vi "Init Scene.vi"(8 "error in (no error)":errorcluster, 11 "SceneGraph Refnum":refnum<vi>) -> (0 "error out":errorcluster, 3 "Voronoi Grid Object":refnum<vi>)   [LabVIEW 2023]
doc: "Initialize the overall scene by setting camera parameters and creating the object for the Voronoi surface."
uses:
  <vilib>/Utility/miscctls.llb/LV3DPointTypeDef.ctl
  <vilib>/picture/3D Picture Control/Object/Create Object (name).vi
  <vilib>/picture/3D Picture Control/NI_3D Picture Control.lvlib
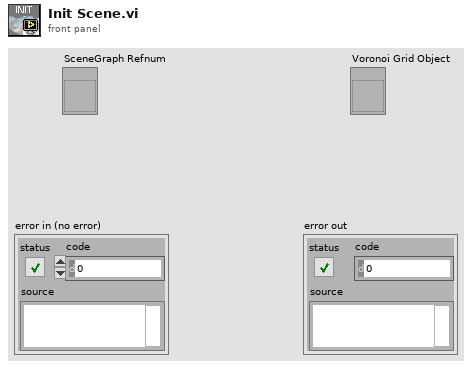
[diagram p1: front panel]
types:
  T1 = enum16{"None", "Spherical", "Flying", "Oriented"}
  T2 = typedef "LV3DPointTypeDef.ctl" = cluster{"X":sgl, "Y":sgl, "Z":sgl}
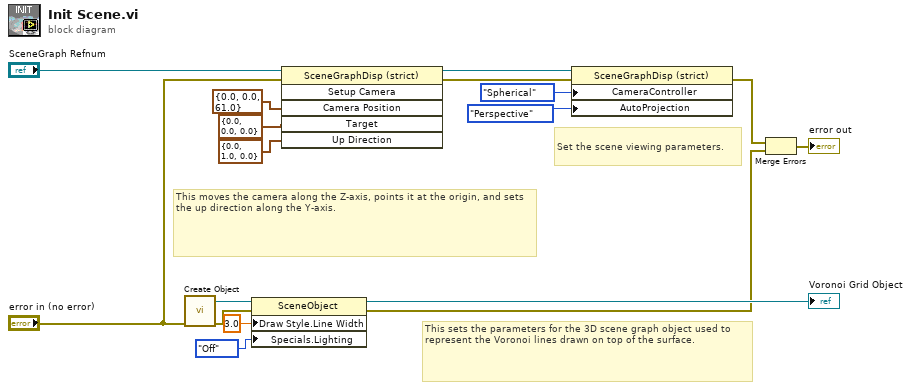
[diagram p0: block diagram]
diagram:
  # "This sets the parameters for the 3D scene graph object used to represent the Voronoi lines drawn on top of the surface."
  # "This moves the camera along the Z-axis, points it at the origin, and sets the up direction along the Y-axis."
  # "Set the scene viewing parameters."
  n1 = call-poly <vilib>:"Create Object.vi"("error in (no error)"="error in (no error)") -> ("error out"=w6:errorcluster, "Scene:New Object"=w16:refnum<vi>)  [unwired: 9 in]
  n2 = property class="SceneObject"(reference=w16, error in=w6, "Draw Style.Line Width"=sgl 3.0 ("Draw Style:Line Width"), "Specials.Lighting"=enum16{"Inherit Value", "Off", "On"}."Off" ("Specials:Lighting")) -> (reference out=→"Voronoi Grid Object":refnum<vi>, error out=w2:errorcluster)
  n3 = invoke on="Invoke Node" class="SceneGraphDisp (strict)" method="Setup Camera"(reference="SceneGraph Refnum", error in="error in (no error)", "Camera Position"=T2 {"X"=0.0, "Y"=0.0, "Z"=61.0}, "Target"=T2 {"X"=0.0, "Y"=0.0, "Z"=0.0}, "Up Direction"=T2 {"X"=0.0, "Y"=1.0, "Z"=0.0}) -> (reference out=w8:refnum<vi>, error out=w5:errorcluster)  [unwired: 1 in, 4 out]
  n4 = property on="Property Node" class="SceneGraphDisp (strict)"(reference=w8, error in=w5, "CameraController"=T1."Spherical" ("Camera Controller:Type"), "AutoProjection"=enum16{"None", "Perspective", "Orthographic"}."Perspective" ("Automatic Projection Mode")) -> (error out=w3:errorcluster)  [unwired: 1 out]
  n5 = Merge Errors(w3, w2) -> (→"error out":errorcluster)
